vi "data.vi"(7 "LabVIEW Web Service Request":refnum<class "Web Request.lvclass">) -> ()   [LabVIEW 2021]
uses:
  <vilib>/wsapi/Web Request.lvclass
  3c4a661f-b223-40ff-afd8-50993ca65a23.vi
  f6cf2a47-77fc-487e-85e6-73694e6b0073.vi
  <vilib>/JDP Science/JSONtext/Variant to JSON Text.vi
  <userlib>/S2 Labs/Error Reporting/ER Global.vi
  <userlib>/S2 Labs/Error Reporting/Error Reporting Class/subVIs/Report Error.vi
  <vilib>/JDP Science/JSONtext/LVClass Serializer/JSONtext LVClass Serializer.lvclass
  <userlib>/S2 Labs/Module Framework/Modules/Base/Module.lvclass
panel:
  # "Use the Web Service Request input terminal to call the VIs on the Web Services palette. Do not remove it from the connector pane unless you don't need access to the palette."
  # "Each additional control wired to the connector pane will be available as an input in the URL. To include an indicator in terminal-mode output (the default setting), it must also be wired to the connector pane."
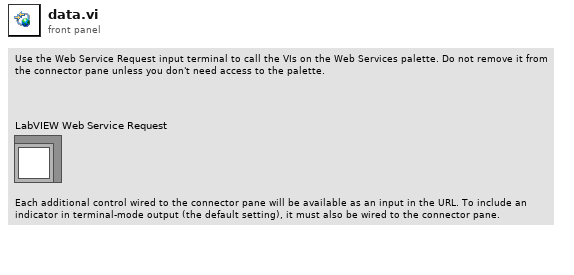
[diagram p1: front panel]
types:
  T1 = cluster{"module":string, "channel":string, "Value":dbl, "Time Stamp":timestamp, "Variant":cluster{"var":variant}, "variant value?":bool}[]
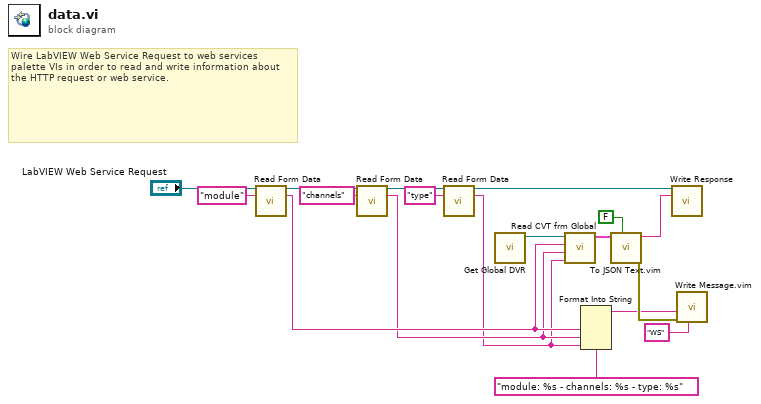
[diagram p0: block diagram]
diagram:
  # "Wire LabVIEW Web Service Request to web services palette VIs in order to read and write information about the HTTP request or web service."
  n1 = call <vilib>:"Read Form Data.vi"("LabVIEW Web Service Request"="LabVIEW Web Service Request", "key"="module") -> ("LabVIEW Web Service Request out"=w8:refnum<class "Web Request.lvclass">, "value"=w3:string)  [unwired: 10 in, 2 out]
  n2 = call <vilib>:"Read Form Data.vi"("LabVIEW Web Service Request"=w8, "key"="channels") -> ("LabVIEW Web Service Request out"=w6:refnum<class "Web Request.lvclass">, "value"=w2:string)  [unwired: 10 in, 2 out]
  n3 = call <vilib>:"Read Form Data.vi"("LabVIEW Web Service Request"=w6, "key"="type") -> ("LabVIEW Web Service Request out"=w7:refnum<class "Web Request.lvclass">, "value"=w1:string)  [unwired: 10 in, 2 out]
  n4 = call <userlib>:"Get Global DVR.vi"() -> ("Global DVR"=w18:refnum<data-value>)  [unwired: 11 in]
  n5 = call <userlib>:"Read CVT frm Global.vi"("Type"=w1, "Channels"=w2, "Module"=w3, "Global DVR"=w18) -> ("Data"=w17:T1)  [unwired: 7 in]
  n6 = Format Into String(format string="module: %s - channels: %s - type: %s", w3, w2, w1) -> (resulting string=w11:string)  [unwired: 2 in, 1 out]
  n7 = call "To JSON Text.vim"("enable LabVIEW extensions? (T)"=FALSE, "Anything"=w17) -> ("error out"=w15:errorcluster, "<JSON>"=w13:string)  [unwired: 8 in]
  n8 = call <vilib>:"Write Response.vi"("LabVIEW Web Service Request"=w7, "response string"=w13) -> ()  [unwired: 12 in, 2 out]
  n9 = call "Write Message.vim"("Message Tag"="WS", "error in (no error)"=w15, "Message (string)"=w11) -> ()  [unwired: 8 in, 1 out]
